vi "GetBarHeight.vi"(8 "error in (no error)":errorcluster, 11 "Code128 in":refnum<class "Code128.lvclass">) -> (0 "error out":errorcluster, 2 "Bar Height":u8=25, 3 "Code128 out":refnum<class "Code128.lvclass">)   [LabVIEW 2013, in "BarCodes.lvlib" / "Code128.lvclass"]
uses:
  Code128.lvclass
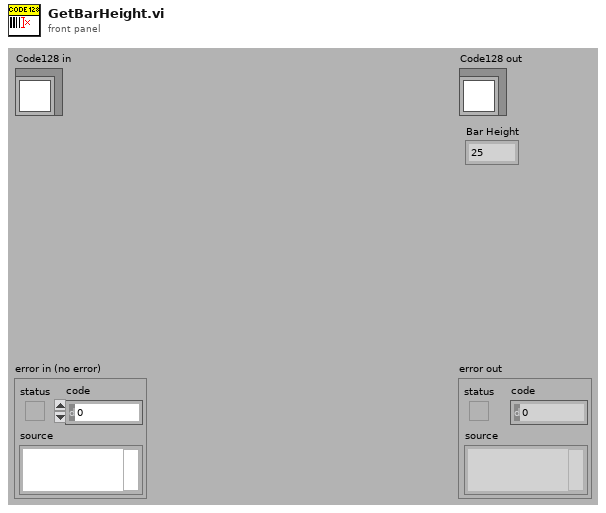
[diagram p1: front panel]
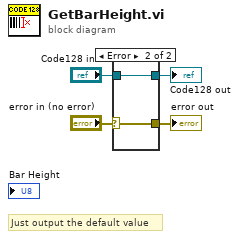
[diagram p0: block diagram]
diagram:
  # "Just output the default value"
  n1 = case shown="Error" "error in (no error)" {
    selector: "error in (no error)" -> [w6 w8]
    tunnel: [w6 w8] -> w3
    tunnel: "Code128 in" -> [w5 w7]
    tunnel: [w5 w7] -> w1
    frame No Error {
    }
    frame Error {
    }
  }
  "error out" <- w3
  "Code128 out" <- w1
